vi "Publish.vi"(8 "error in (no error)":errorcluster, 9 "Payload":variant, 10 "Topic Name (empty: Payload name)":string, 11 "Client in":refnum<class "Client.lvclass">) -> (0 "error out":errorcluster, 3 "Client out":refnum<class "Client.lvclass">)   [LabVIEW 2013, in "MQTT Server.lvlib" / "Client.lvclass"]
uses:
  Client.lvclass
  <vilib>/LabVIEW Open Source Project/Configuration Manager/Serializer/Serializer.lvclass
  Client.lvclass/Client.ctl
  <vilib>/LabVIEW Open Source/Data Manipulation/TypeDescriptor/TypeDescriptor_GetName.vi
  <vilib>/LabVIEW Open Source/Data Manipulation/TypeDescriptor/TypeDescriptor_GetPString.vi
  Server/Session/Session.lvclass
  Control Packets/PUBLISH/PUBLISH.lvclass
  <vilib>/LabVIEW Open Source/Data Manipulation/Variant/OpenVariant.lvlib
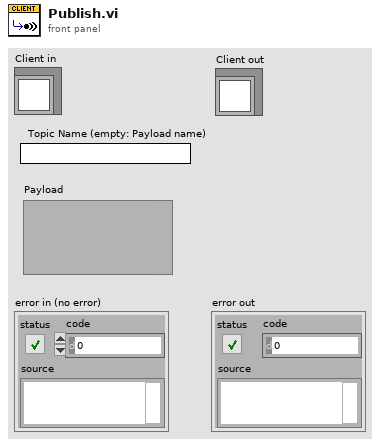
[diagram p1: front panel]
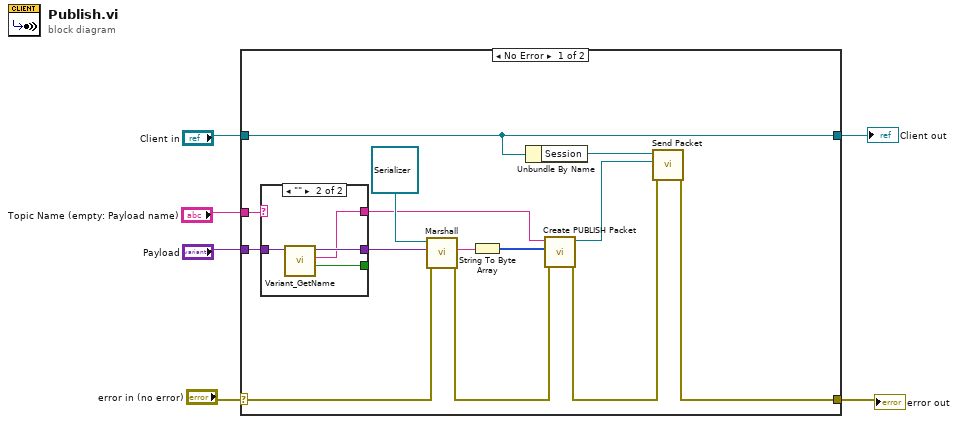
[diagram p0: block diagram]
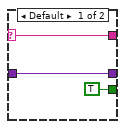
[diagram p2: hidden frame]
diagram:
  n1 = case shown="No Error" "error in (no error)" {
    selector: "error in (no error)" -> [w12 w29]
    tunnel: [w8 w29] -> w1
    tunnel: [w10 w28] -> w2
    tunnel: "Client in" -> [w10 w28]
    tunnel: "Payload" -> [w17 _]
    tunnel: "Topic Name (empty: Payload name)" -> [w15 _]
    frame No Error {
      n2 = case shown="\"\"" w15 {
        selector: w15 -> [w23 _]
        tunnel: w17 -> [w22 w27]
        tunnel: [w22 w26] -> w16
        tunnel: [w23 w25] -> w14
        tunnel: [TRUE ("found") w24] -> _
        frame Default {
        }
        frame "" {
          n3 = call <vilib>:"Variant_GetName.vi"("Variant"=w27) -> ("found"=w24:bool, "Name"=w25:string, "Variant dup"=w26:variant)  [unwired: 8 in]
        }
      }
      n4 = call-dynamic "Marshall.vi"("error in (no error)"=w12, "Variant"=w16, "Serializer in"=refnum<class "Serializer.lvclass"> refnum) -> ("error out"=w13:errorcluster, "String"=w20:string)  [unwired: 6 in, 1 out]
      n5 = String To Byte Array(string=w20) -> (unsigned byte array=w19:u8[])
      n6 = Unbundle By Name(w10) -> ("Session"=w11:refnum<class "Session.lvclass">)
      n7 = call "Create PUBLISH Packet.vi"("error in (no error)"=w13, "Payload"=w19, "Topic Name"=w14) -> ("error out"=w9:errorcluster, "PUBLISH"=w7:refnum<class "PUBLISH.lvclass">)  [unwired: 6 in, 1 out]
      n8 = call "Send Packet.vi"("error in (no error)"=w9, "Packet"=w7, "Session in"=w11) -> ("error out"=w8:errorcluster)  [unwired: 6 in, 2 out]
    }
    frame Error {
    }
  }
  "error out" <- w1
  "Client out" <- w2
